vi "servo.vi"() -> ()   [LabVIEW 2018]
uses:
  <vilib>/Rock Robotics/SystemInterfaces/DIO/FPGA_DIOPWMChannel.ctl
panel:
  in  "stop":bool
  in  "Position":dbl(slide) scale=0.0..1.0
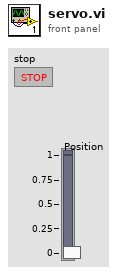
[diagram p1: front panel]
types:
  T1 = typedef "FPGA_DIOPWMChannel.ctl" = enum8{"PWM 0", "PWM 1", "PWM 2", "PWM 3", "PWM 4", "PWM 5", "PWM 6", "PWM 7", "PWM 8", "PWM 9", "PWM MXP 0", "PWM MXP 1", "PWM MXP 2", "PWM MXP 3", "PWM MXP 4", "PWM MXP 5", "PWM MXP 6", "PWM MXP 7", "PWM MXP 8", "PWM MXP 9", "Invalid"}
  T2 = typedef "WPI_ServoDeviceRef.ctl" = cluster{"DeviceStatus":errorcluster, "PWM Channel":T1, "DeadBand":T3}
  T3 = typedef "WPI_PWMDeadband.ctl" = cluster{"Name":string, "maxPositivePwm":i32, "minPositivePwm":i32, "centerPwm":i32, "maxNegativePwm":i32, "minNegativePwm":i32, "angularRange":u16}
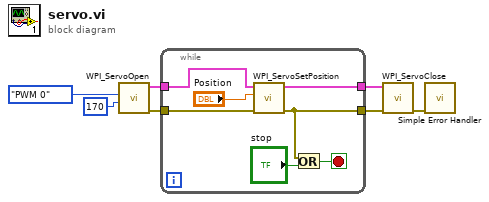
[diagram p0: block diagram]
diagram:
  n1 = call <vilib>:"WPI_ServoOpen.vi"("Angular Range"=u16 170, "PWM Channel"=FPGA_DIOPWMChannel."PWM 0") -> ("error out"=w3:errorcluster, "ServoDeviceRef"=w5:T2)  [unwired: 8 in]
  n2 = while {
    tunnel: w5 -> [w14]
    tunnel: [w10] -> w4
    tunnel: w3 -> [w9]
    tunnel: [w8] -> w2
    stop <- w11 stop-if-true
    n3 = call <vilib>:"WPI_ServoSetPosition.vi"("error in (no error)"=w9, "Position"="Position", "ServoDeviceRef"=w14) -> ("error out"=w8:errorcluster, "ServoDeviceRef"=w10:T2)  [unwired: 7 in]
    n4 = Or(x=w8, y="stop") -> (x .or. y?=w11:bool)
  }
  n5 = call <vilib>:"WPI_ServoClose.vi"("error in (no error)"=w2, "ServoDeviceRef"=w4) -> ("error out"=w1:errorcluster)  [unwired: 9 in]
  n6 = call <vilib>:"Simple Error Handler.vi"("error in (no error)"=w1) -> ()  [unwired: 4 in, 5 out]
